vi "Untitled 4.vi"() -> ()   [LabVIEW 2022 SP3]
uses:
  <vilib>/addons/control/pid/pid.llb/PID Gain Schedule (DBL).vi
  <vilib>/addons/control/pid/pid.llb/PID (DBL).vi
  <vilib>/addons/control/pid/NI_PID_pid.lvlib
panel:
  out "PRESSURE":dynamicdata(graph)
  in  "stop":bool
  in  "SP":dbl
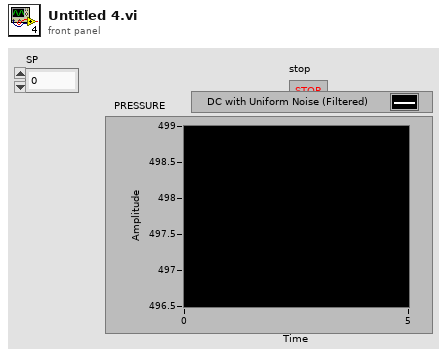
[diagram p1: front panel]
types:
  T1 = cluster{"proportional gain (Kc)":dbl, "integral time (Ti, min)":dbl, "derivative time (Td, min)":dbl}
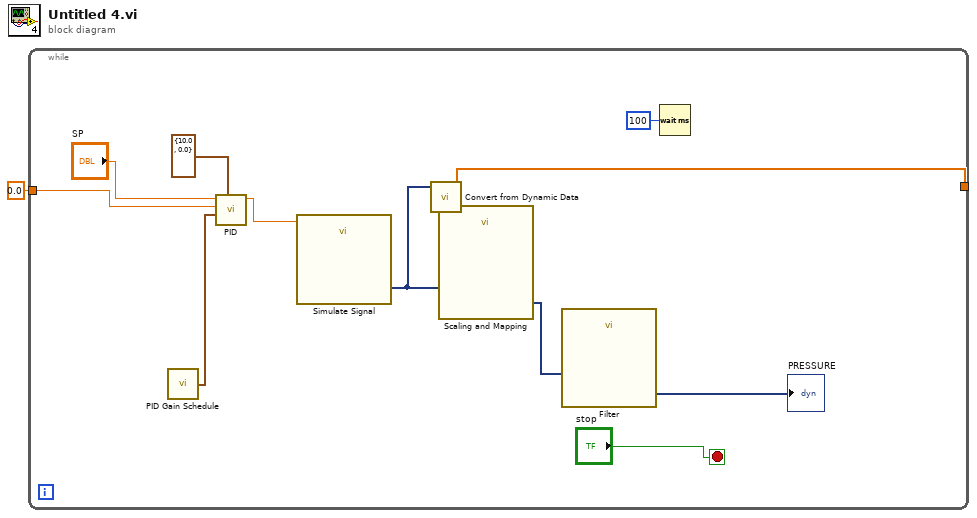
[diagram p0: block diagram]
diagram:
  n1 = while {
    tunnel: 0.0 ("process variable") -> [w8]
    tunnel: [w3] -> _
    stop <- "stop" stop-if-true
    n2 = call-poly <vilib>:"PID Gain Schedule.vi"() -> ("PID gains out"=w11:T1)  [unwired: 4 in, 1 out]
    n3 = call-poly <vilib>:"PID.vi"("output range"=cluster{"output high":dbl, "output low":dbl} {"output high"=10.0, "output low"=0.0}, "PID gains"=w11, "process variable"=w8, "setpoint"="SP") -> ("output"=w10:dbl)  [unwired: 6 in, 1 out]
    n4 = call "Simulate Signal"("Offset"=w10) -> ("DC with Uniform Noise"=w4:dynamicdata)  [unwired: 13 in, 1 out]
    n5 = call "Convert from Dynamic Data"("Dynamic Data Type"=w4) -> ("Array"=w3:dbl[])  [unwired: 3 in]
    n6 = call "Scaling and Mapping"("Signals"=w4) -> ("Scaled Signals"=w7:dynamicdata)  [unwired: 9 in, 1 out]
    n7 = call "Filter"("Signal"=w7) -> ("Filtered Signal"=→"PRESSURE":dynamicdata)  [unwired: 9 in, 1 out]
    n8 = Wait (ms)(milliseconds to wait=u32 100) -> ()  [unwired: 1 out]
  }
